vi "Set Write Options.vi"(8 "error in (no error)":errorcluster, 9 "dwFlags":u32, 10 "Compression Level":u32=6, 11 "BLF File In":refnum<class "Read Write BLF.lvclass">) -> (0 "error out":errorcluster, 3 "BLF File Out":refnum<class "Read Write BLF.lvclass">)   [LabVIEW 2015, in "Read Write BLF.lvclass"]
doc: "This VI will set write options for a BLF file such as the file compression level which defaults to 6 out of 10 where 10 is higher compression and 0 is none.\n\n-------------\nBrian Hoover (Hooovahh)"
uses:
  Read Write BLF.lvclass
  Read Write BLF.lvclass/Read Write BLF.ctl
  <vilib>/Utility/error.llb/Error Cluster From Error Code.vi
  <vilib>/Utility/libraryn.llb/Check if File or Folder Exists.vi
  <vilib>/Utility/file.llb/Application Directory.vi
  <vilib>/ErrorRing/Error Ring.xnode
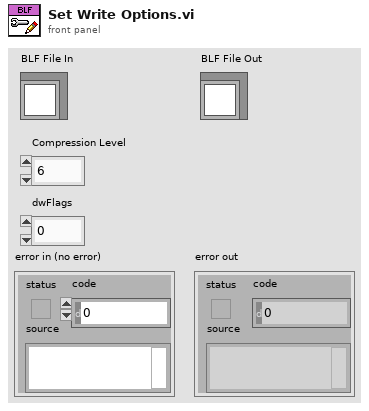
[diagram p1: front panel]
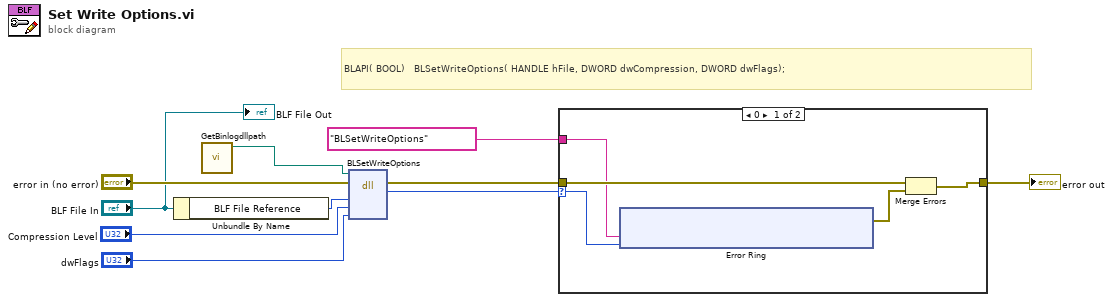
[diagram p0: block diagram]
diagram:
  # "BLAPI( BOOL)   BLSetWriteOptions( HANDLE hFile, DWORD dwCompression, DWORD dwFlags);"
  n1 = Unbundle By Name("BLF File In") -> ("BLF File Reference"=w2:u32)
  n2 = call "GetBinlogdllpath.vi"() -> ("dup path"=w1:path)  [unwired: 11 in]
  n3 = dll-call lib="PTH2Tabs E自开发软件X-CAN项目X-CAN离线分析平台 V2.3.1BLFbinlog.*" fn="BLSetWriteOptions"(path in=w1, error in="error in (no error)", "hFile"=w2, "dwCompression"="Compression Level", "dwFlags"="dwFlags") -> (error out=w5:errorcluster, "返回类型"=w4:i32)  [unwired: 4 in, 1 out]
  n4 = case shown="0" w4 {
    selector: w4 -> [w13 _]
    tunnel: w5 -> [w15 w24]
    tunnel: [w14 w24] -> w6
    tunnel: "BLSetWriteOptions" -> [w12 _]
    frame 0 {
      n5 = xnode "Error Ring"("参数 0"=w12, "参数 1"=w13) -> ("错误输出"=w11:errorcluster)
      n6 = Merge Errors(w15, w11) -> (w14:errorcluster)
    }
    frame Default {
    }
  }
  "error out" <- w6
  "BLF File Out" <- "BLF File In"
